vi "auto_alignment_v2-2.vi"() -> ()   [LabVIEW 2024]
uses:
  O:/DSG/Tyler/EIC/DIRC/daq/automated/Thorlabs.MotionControl.IntegratedStepperMotorsCLI.dll
  Thorlabs.MotionControl.IntegratedStepperMotorsCLI.dll
  O:/DSG/Tyler/EIC/DIRC/daq/automated/Thorlabs.MotionControl.Benchtop.StepperMotorCLI.dll
  Thorlabs.MotionControl.Benchtop.StepperMotorCLI.dll
  301acc45-ca86-4456-a934-959b204451cf.vi
  874d4c17-ce3d-4308-86ed-5be04f0cb30b.vi
  5035e5c4-651a-4bea-8586-5c5be43a7c01.vi
  c928da2b-9bf4-4dff-b90d-86dfb6fa8dbf.vi
  97e29fd1-0a36-40b5-96b6-4bface3040cf.vi
  <vilib>/Array/Sort 2D Array - Pop Stack.vi
  <vilib>/Array/Sort 2D Array - Push Stack.vi
  301acc45-ca86-4456-a934-959b204451cf.vi/269d4b3b-47f5-49e3-8884-44851e4dd9d5.vi
  301acc45-ca86-4456-a934-959b204451cf.vi/6d99389c-673d-4efb-bf33-19b32bcf4cf8.vi
  874d4c17-ce3d-4308-86ed-5be04f0cb30b.vi/269d4b3b-47f5-49e3-8884-44851e4dd9d5.vi
  874d4c17-ce3d-4308-86ed-5be04f0cb30b.vi/6d99389c-673d-4efb-bf33-19b32bcf4cf8.vi
  5035e5c4-651a-4bea-8586-5c5be43a7c01.vi/269d4b3b-47f5-49e3-8884-44851e4dd9d5.vi
  5035e5c4-651a-4bea-8586-5c5be43a7c01.vi/6d99389c-673d-4efb-bf33-19b32bcf4cf8.vi
  c928da2b-9bf4-4dff-b90d-86dfb6fa8dbf.vi/269d4b3b-47f5-49e3-8884-44851e4dd9d5.vi
  c928da2b-9bf4-4dff-b90d-86dfb6fa8dbf.vi/6d99389c-673d-4efb-bf33-19b32bcf4cf8.vi
  97e29fd1-0a36-40b5-96b6-4bface3040cf.vi/269d4b3b-47f5-49e3-8884-44851e4dd9d5.vi
  97e29fd1-0a36-40b5-96b6-4bface3040cf.vi/6d99389c-673d-4efb-bf33-19b32bcf4cf8.vi
  <vilib>/Utility/file.llb/Read Delimited Spreadsheet (string).vi
  <vilib>/Analysis/NI_AALBase.lvlib
panel:
  out "sim_y-range":dbl[](array[numeric])
  out "sim_x-range":dbl[](array[numeric])
  out "sim_max":dbl[](array[numeric])
  out "Array":string[](array[string])
  in  "early-stop":bool
  out "state":string
  out "nPts":dbl
  out "pt-history":dbl[][](array[numeric])
  out "real-mode":bool
  out "sim-iCorr":dbl[](array[numeric])
  out "sim-pdy":dbl[](array[numeric])
  out "sim-pdx":dbl[](array[numeric])
  out "sim-data":dbl[][](array[numeric])
  out "Final Location":dbl[](array[numeric])
  out "x_c":dbl[](array[numeric])
  out "x_e":dbl[](array[numeric])
  out "x_r":dbl[](array[numeric])
  out "timeout":bool
  out "se_done":bool
  in  "se_goal":dbl=0.04
  out "squared_error":dbl
  out "x_o":dbl[](array[numeric])
  in  "xStart":dbl=265.0 format="%#_13g"
  in  "yStart":dbl=127.5 format="%#_13g"
  in  "stage-refs":T1
  in  "nSamples":dbl=10.0 caption="# Samples"
  in  "NM-params":T2={"alpha"=1.0, "gamma"=2.0, "rho"=0.5, "sigma"=0.5, "simplex L"=0.5}
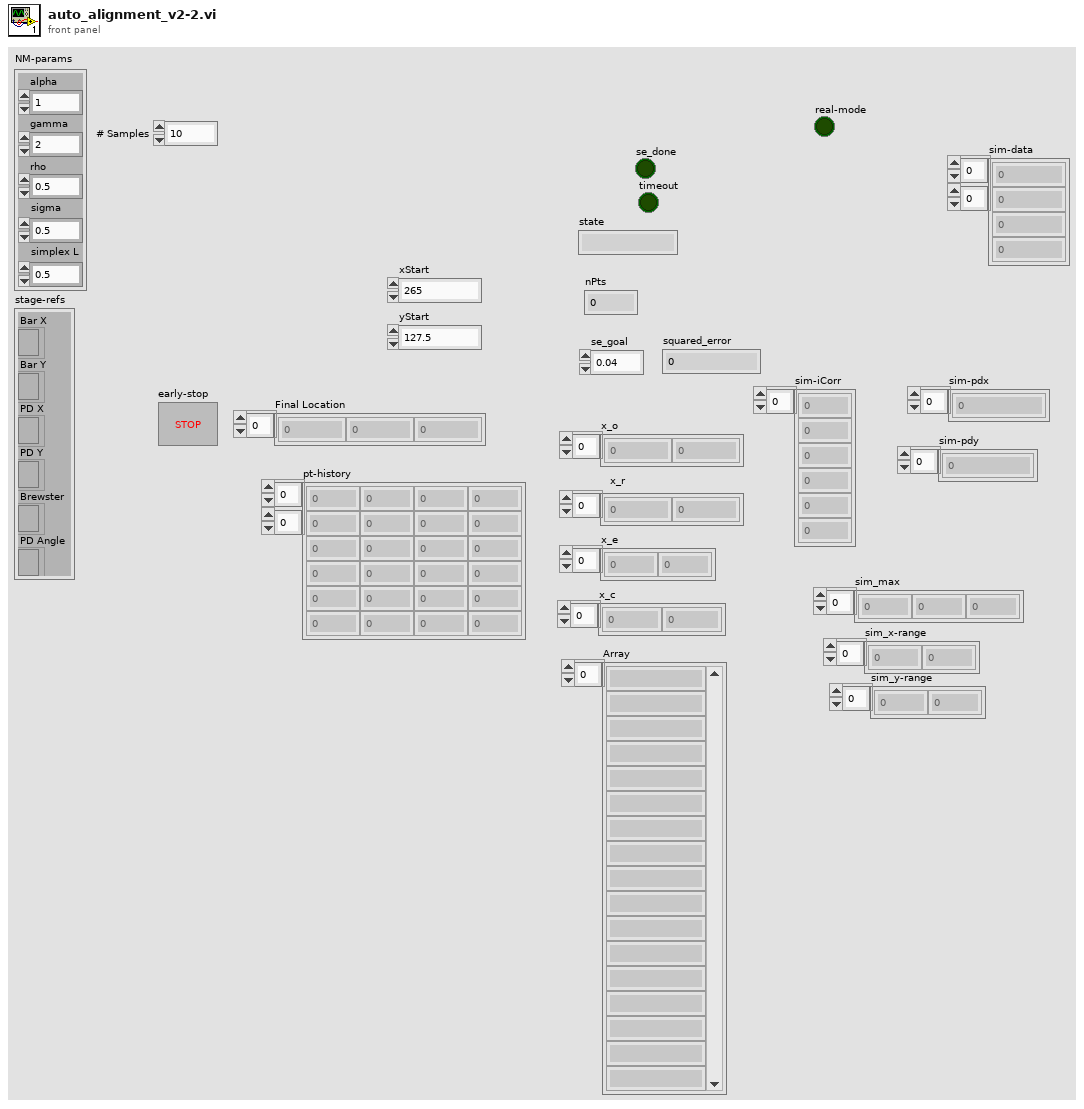
[diagram p1: front panel]
types:
  T1 = cluster{"Bar X":refnum<k24>, "Bar Y":refnum<k24>, "PD X":refnum<k24>, "PD Y":refnum<k24>, "Brewster":refnum<k24>, "PD Angle":refnum<k24>}
  T2 = cluster{"alpha":dbl, "gamma":dbl, "rho":dbl, "sigma":dbl, "simplex L":dbl}
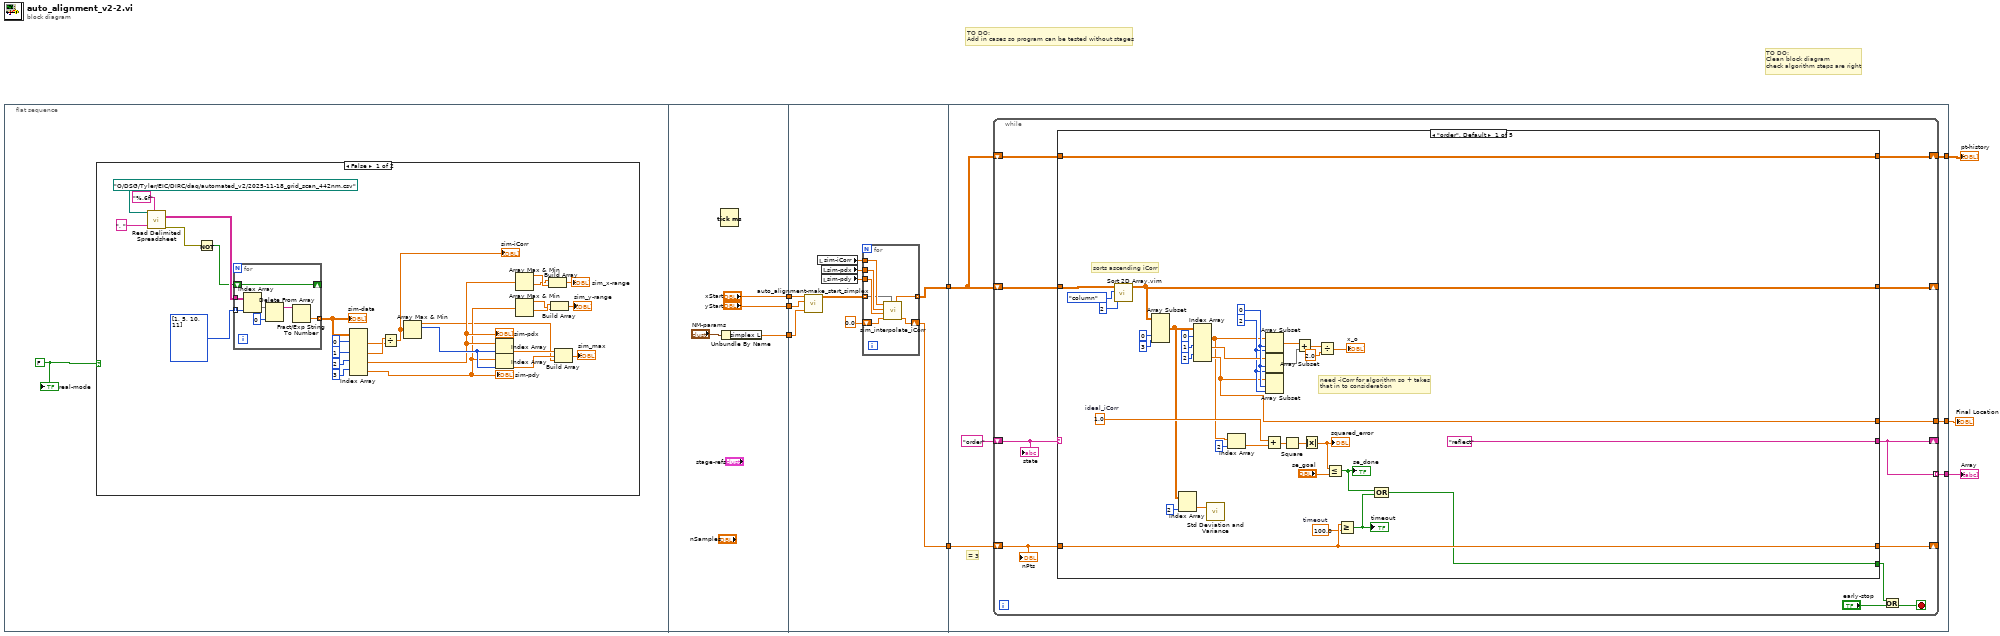
[diagram p0: block diagram]
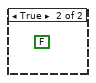
[diagram p2: hidden frame]
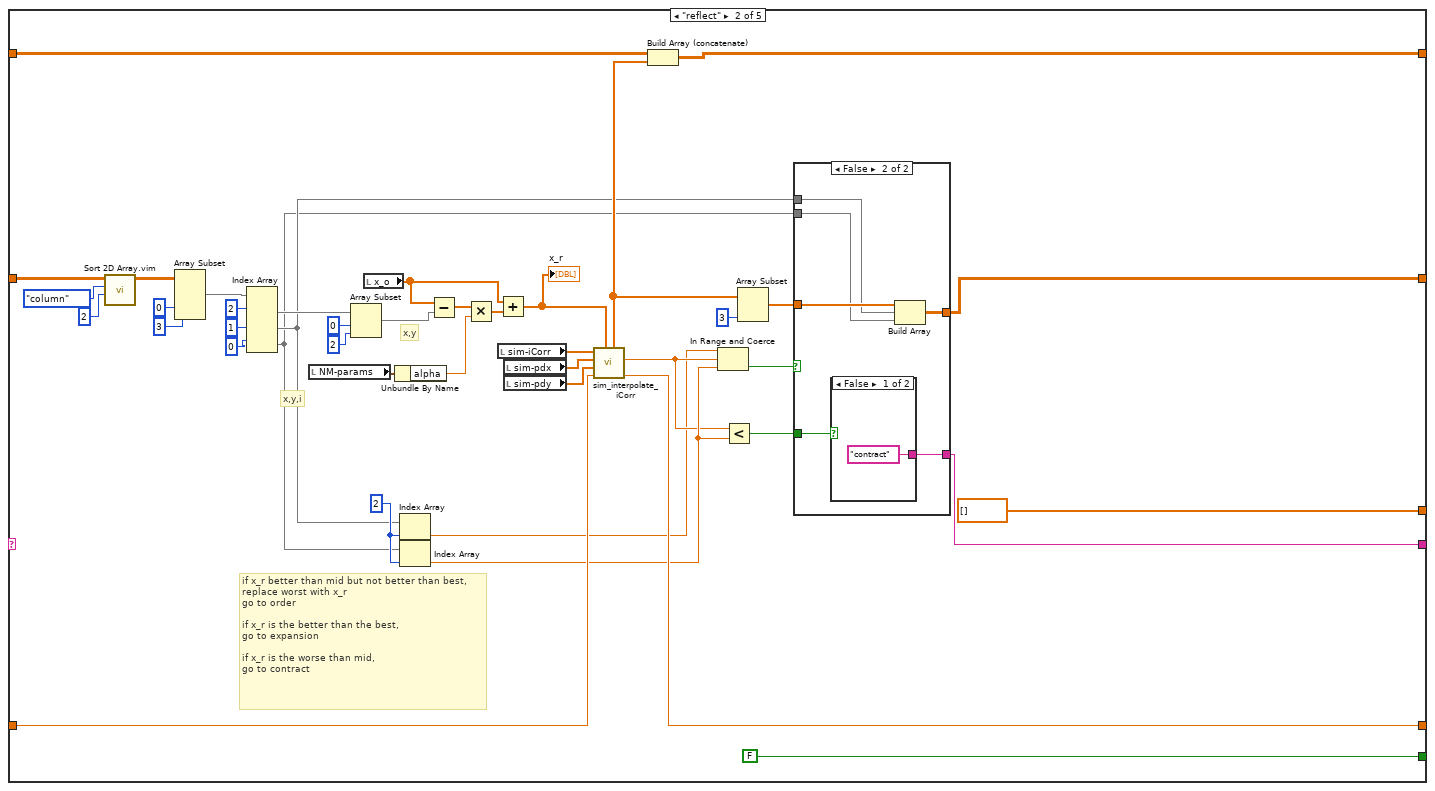
[diagram p3: hidden frame]
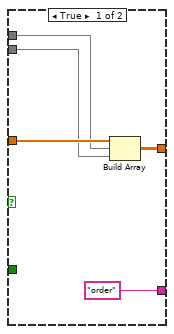
[diagram p4: hidden frame]
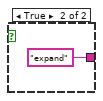
[diagram p5: hidden frame]
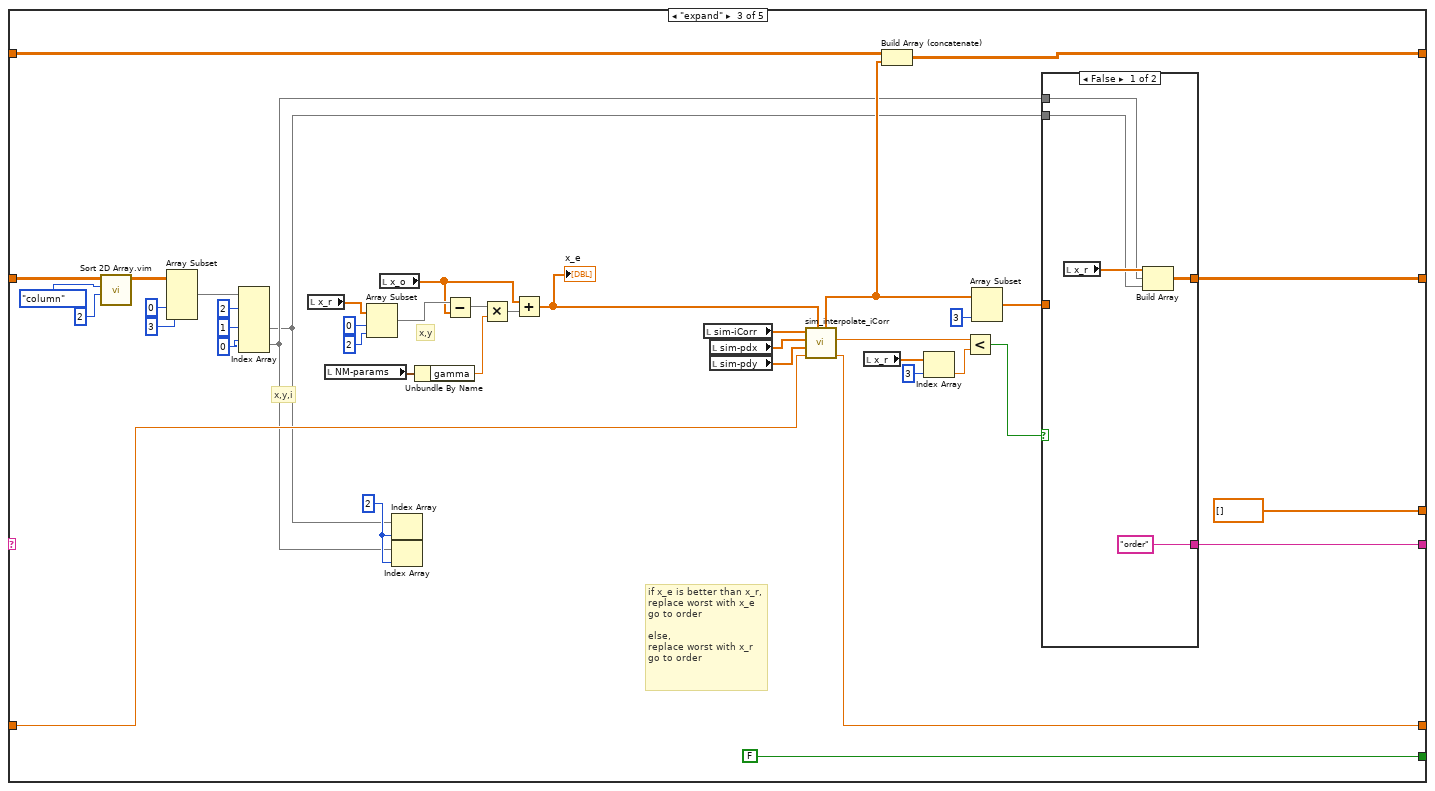
[diagram p6: hidden frame]
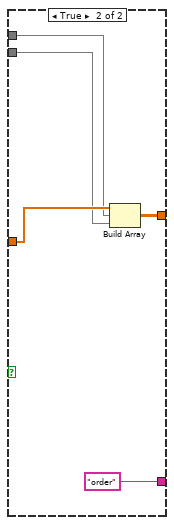
[diagram p7: hidden frame]
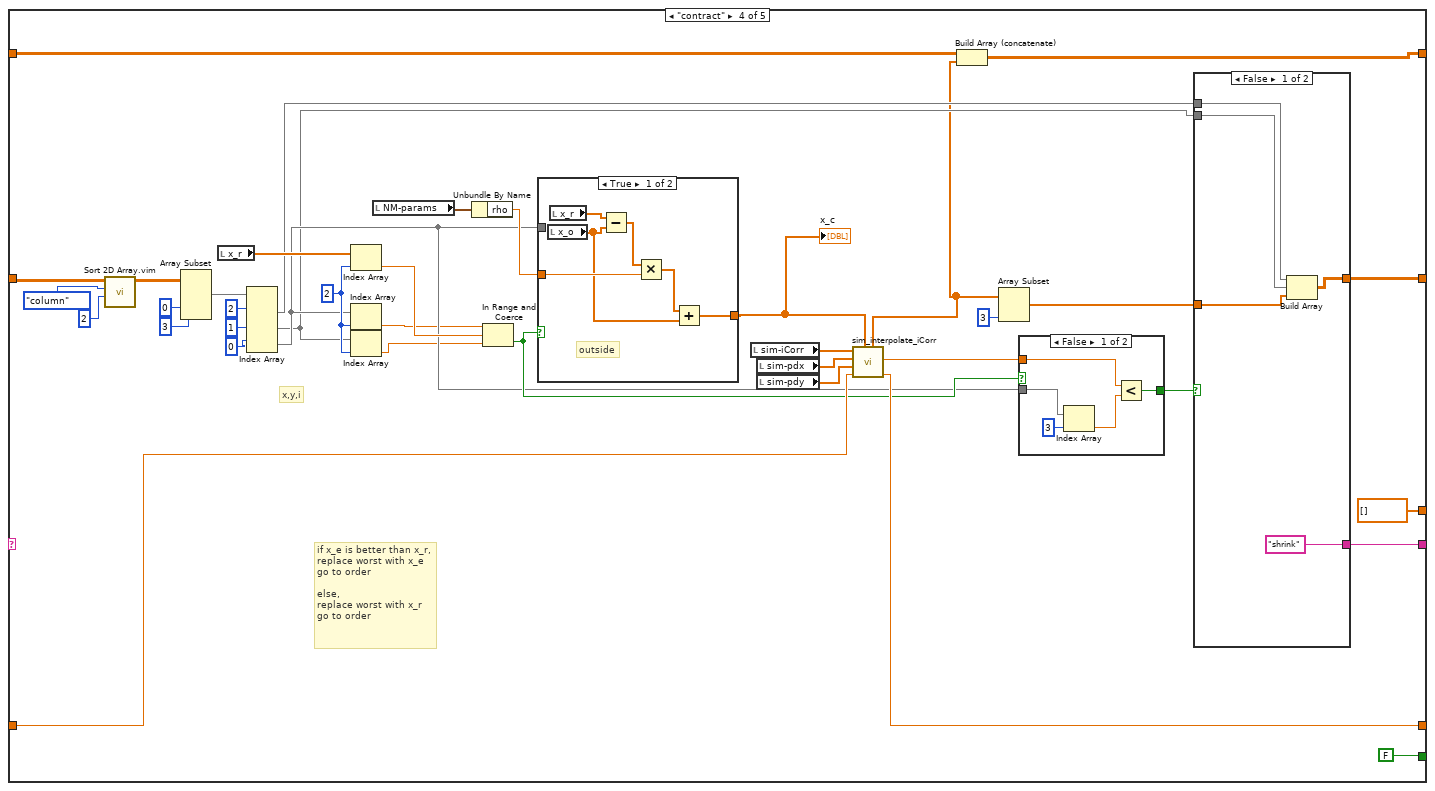
[diagram p8: hidden frame]
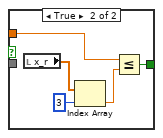
[diagram p9: hidden frame]
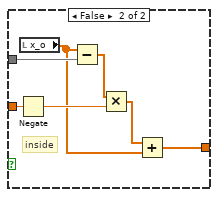
[diagram p10: hidden frame]
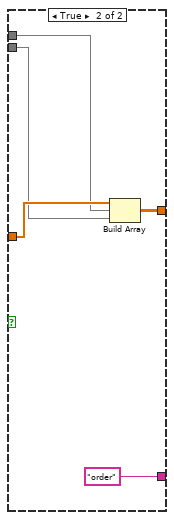
[diagram p11: hidden frame]
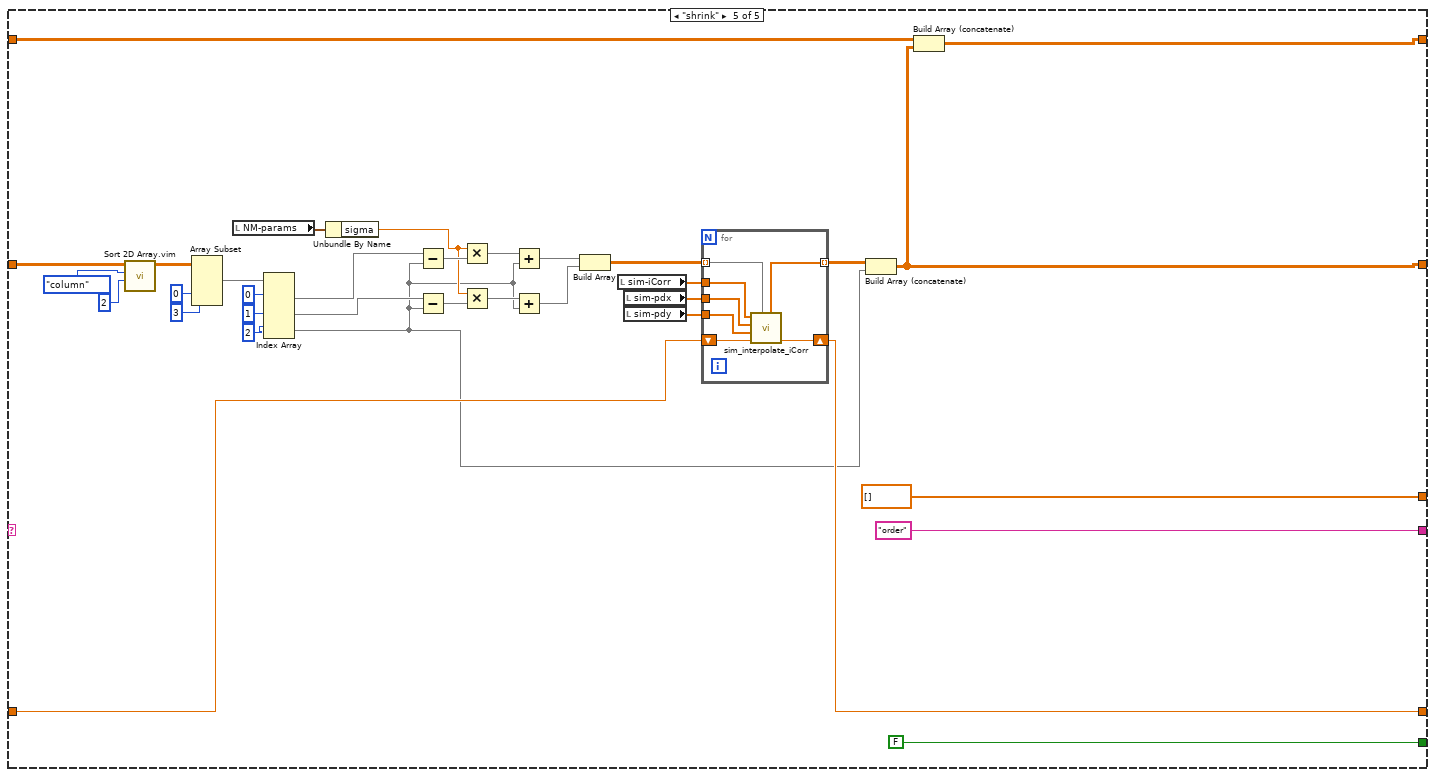
[diagram p12: hidden frame]
diagram:
  # "TO DO:\nClean block diagram\ncheck algorithm steps are right"
  # "TO DO:\nAdd in cases so program can be tested without stages"
  n1 = flat-sequence {
    tunnel: ["xStart"] -> w8
    tunnel: ["yStart"] -> w7
    tunnel: [w45] -> w6
    tunnel: [w58] -> w2
    tunnel: [w57] -> w1
    tunnel: w6 -> [w56]
    tunnel: w7 -> [w55]
    tunnel: w8 -> [w54]
    tunnel: w2 -> [w69]
    tunnel: w1 -> [w70]
    tunnel: [w68] -> w5
    tunnel: [w67] -> w4
    tunnel: [w66] -> w3
    frame #0 {
      w9 = FALSE
      n2 = case shown="False" w9 {
        frame False {
          n3 = call-poly <vilib>:"Read Delimited Spreadsheet.vi"("file path (dialog if empty)"=path "O:/DSG/Tyler/EIC/DIRC/daq/automated_v2/2025-11-18_grid_scan_442nm.csv", "format (%s)"="%.6f" ("format (%.3f)"), "delimiter (\\t)"=", " ("delimiter (\\t)")) -> ("all rows"=w33:string[][], "error out"=w35:errorcluster)  [unwired: 7 in, 4 out]
          n4 = Not(x=w35) -> (.not. x?=w31:bool)
          n5 = for {
            tunnel: i32[] [1, 5, 10, 11] -> [w43] mode=indexing
            tunnel: w33 -> [w44]
            shift-right: [w42] -> _
            shift-left: w31 -> [w42]
            tunnel: [w38] -> w24 mode=indexing
            n6 = Index Array(array=w44, index (col)=w43) -> (element=w41:string[])  [unwired: 1 in]
            n7 = Delete From Array(array=w41, index=0) -> (array with subset deleted=w39:string[])  [unwired: 1 in, 1 out]
            n8 = Fract/Exp String To Number(string=w39) -> (number=w38:dbl[])  [unwired: 3 in, 1 out]
          }
          "sim-data" <- w24
          n9 = Index Array(array=w24, index (row) #1=0 ("index"), index (row) #2=1 ("index (row)"), index (row) #3=2 ("index (row)"), index (row) #4=3 ("index (row)")) -> (element #1=w25:dbl[], element #2=w26:dbl[], element #3=w19:dbl[], element #4=w18:dbl[])  [unwired: 4 in]
          "sim-pdx" <- w19
          "sim-pdy" <- w18
          n10 = Divide(x=w26, y=w25) -> (x/y=w10:dbl[])
          "sim-iCorr" <- w10
          n11 = Array Max & Min(array=w10) -> (max value=w11:dbl, max index (indices)=w23:i32)  [unwired: 2 out]
          n12 = Index Array(array=w19, index=w23) -> (element=w22:dbl)
          n13 = Index Array(array=w18, index=w23) -> (element=w21:dbl)
          n14 = Array Max & Min(array=w19) -> (max value=w17:dbl, min value=w16:dbl)  [unwired: 2 out]
          n15 = Array Max & Min(array=w18) -> (max value=w13:dbl, min value=w15:dbl)  [unwired: 2 out]
          n16 = Build Array(w16, w17) -> (→"sim_x-range":dbl[])
          n17 = Build Array(w15, w13) -> (→"sim_y-range":dbl[])
          n18 = Build Array(w22, w21, w11) -> (→"sim_max":dbl[])
        }
        frame True {
          (unwired) FALSE
        }
      }
      "real-mode" <- w9
    }
    frame #1 {
      n19 = Tick Count (ms)() -> ()  [unwired: 1 out]
      n20 = Unbundle By Name("NM-params") -> ("simplex L"=w45:dbl)
    }
    frame #2 {
      n21 = call "auto_alignment-make_start_simplex.vi"("L"=w56, "yStart"=w55, "xStart"=w54) -> ("Array"=w53:dbl[][])  [unwired: 8 in]
      n22 = local read "sim-iCorr"() -> (w51:dbl[])
      n23 = local read "sim-pdx"() -> (w49:dbl[])
      n24 = local read "sim-pdy"() -> (w50:dbl[])
      n25 = for {
        shift-right: [w60] -> w57
        shift-left: 0.0 -> [w59]
        tunnel: w53 -> [w62] mode=indexing
        tunnel: [w61] -> w58 mode=indexing
        tunnel: w51 -> [w65]
        tunnel: w50 -> [w63]
        tunnel: w49 -> [w64]
        n26 = call "sim_interpolate_iCorr.vi"("point in"=w62, "nPts in"=w59, "sim-pdy"=w63, "sim-pdx"=w64, "sim-iCorr"=w65) -> ("nPts out"=w60:dbl, "measured-point out"=w61:dbl[])  [unwired: 4 in, 1 out]
      }
    }
    frame #3 {
      # "= 3"
      n27 = while {
        shift-right: [w77] -> w67
        shift-left: w69 -> [w82]
        shift-right: [w78] -> _
        shift-left: w69 -> [w81]
        shift-right: [w72] -> _
        shift-left: "order" -> [w83]
        shift-right: [w79] -> _
        shift-left: w70 -> [w80]
        tunnel: [w76] -> w68
        tunnel: [w72] -> w66 mode=indexing
        stop <- w74 stop-if-true
        n28 = case shown="\"order\", Default" w83 {
          tunnel: w82 -> [w105 w143 w200 w254 w311]
          tunnel: w81 -> [w104 w121 w176 w229 w298]
          tunnel: ["reflect" w139 w196 w251 "order"] -> w72
          tunnel: w80 -> [w95 w145 w202 w256 w312]
          tunnel: [w95 w144 w201 w255 w309] -> w79
          tunnel: [w96 w140 w197 w252 w306] -> w78
          tunnel: [w91 FALSE FALSE FALSE FALSE] -> w73
          tunnel: [w105 w142 w199 w253 w310] -> w77
          tunnel: [w90 dbl[] [] dbl[] [] dbl[] [] dbl[] []] -> w76
          frame "order", Default {
            w94 = 100.0  # timeout
            w101 = 1.0  # ideal_iCorr
            w110 = 2 ("length")
            w112 = 0 ("index")
            # "need -iCorr for algorithm so + takes\nthat in to consideration"
            # "sorts ascending iCorr"
            n29 = call "Sort 2D Array.vim"("index"=2, "dimension to index (column)"=enum16{"column", "row"}."column", "2D array"=w104) -> ("sorted 2D array"=w96:dbl[][])  [unwired: 7 in, 1 out]
            n30 = Array Subset(array=w96, index (col)=0 ("index"), length (col)=3 ("length")) -> (w86:dbl[][])  [unwired: 2 in]
            n31 = Index Array(array=w86, index (col)=2 ("disabled index (col)")) -> (element=w84:dbl[])  [unwired: 1 in]
            n32 = Index Array(array=w86, index (row) #1=0 ("index (row)"), index (row) #2=1 ("index (row)"), index (row) #3=2 ("index (row)")) -> (element #1=w87:dbl[], element #2=w111:dbl[], element #3=w90:dbl[])  [unwired: 3 in]
            n33 = call <vilib>:"Std Deviation and Variance.vi"("X"=w84) -> ()  [unwired: 1 in, 3 out]
            n34 = Index Array(array=w87, index=2) -> (element=w102:dbl)
            n35 = Add(x=w101, y=w102) -> (x+y=w100:dbl)
            n36 = Array Subset(array=w87, index=w112, length=w110) -> (w89:dbl[])
            n37 = Array Subset(array=w111, index=w112, length=w110) -> (w88:dbl[])
            n38 = Array Subset(array=w90, index=w112, length=w110) -> ()  [unwired: 1 out]
            n39 = Square(x=w100) -> (x^2=w99:dbl)
            n40 = Add(x=w89, y=w88) -> (x+y=w109:dbl[])
            n41 = Absolute Value(x=w99) -> (abs(x)=w98:dbl)
            "squared_error" <- w98
            n42 = Divide(x=w109, y=2.0) -> (x/y=→"x_o":dbl[])
            n43 = Less Or Equal?(x=w98, y="se_goal") -> (x <= y?=w93:bool)
            "se_done" <- w93
            n44 = Greater Or Equal?(x=w95, y=w94) -> (x >= y?=w92:bool)
            "timeout" <- w92
            n45 = Compound Arithmetic op=OR(w93, w92) -> (w91:bool)
          }
          frame "reflect" {
            w141 = 2 ("index")
            # "x,y"
            # "if x_r better than mid but not better than best, \nreplace worst with x_r\ngo to order\n\nif x_r is the better than the best,\ngo to expansion\n\nif x_r is the worse than mid,\ngo to contract"
            # "x,y,i"
            n46 = call "Sort 2D Array.vim"("index"=2, "dimension to index (column)"=enum16{"column", "row"}."column", "2D array"=w121) -> ("sorted 2D array"=w120:dbl[][])  [unwired: 7 in, 1 out]
            n47 = Array Subset(array=w120, index (col)=0 ("index"), length (col)=3 ("length")) -> (w129:dbl[][])  [unwired: 2 in]
            n48 = Index Array(array=w129, index (row) #1=2 ("index (row)"), index (row) #2=1 ("index (row)"), index (row) #3=0 ("index (row)")) -> (element #1=w155:dbl[], element #2=w128:dbl[], element #3=w127:dbl[])  [unwired: 3 in]
            n49 = local read "NM-params"() -> (w152:T2)
            n50 = Array Subset(array=w155, index=0 ("index (row)"), length=2 ("index (row)")) -> (w151:dbl[])
            n51 = local read "x_o"() -> (w148:dbl[])
            n52 = Unbundle By Name(w152) -> ("alpha"=w149:dbl)
            n53 = Index Array(array=w128, index=w141) -> (element=w131:dbl)
            n54 = Index Array(array=w127, index=w141) -> (element=w134:dbl)
            n55 = Subtract(x=w148, y=w151) -> (x-y=w150:dbl[])
            n56 = Multiply(x=w150, y=w149) -> (x*y=w147:dbl[])
            n57 = Add(x=w148, y=w147) -> (x+y=w146:dbl[])
            "x_r" <- w146
            n58 = local read "sim-iCorr"() -> (w126:dbl[])
            n59 = local read "sim-pdx"() -> (w125:dbl[])
            n60 = local read "sim-pdy"() -> (w124:dbl[])
            n61 = call "sim_interpolate_iCorr.vi"("point in"=w146, "nPts in"=w145, "sim-pdy"=w124, "sim-pdx"=w125, "sim-iCorr"=w126) -> ("nPts out"=w144:dbl, "iCorr out"=w132:dbl, "measured-point out"=w138:dbl[])  [unwired: 4 in]
            n62 = Build Array (concatenate)(w143, w138) -> (w142:dbl[][])
            n63 = In Range and Coerce(upper limit=w131, x=w132, lower limit=w134) -> (In Range?=w133:bool)  [unwired: 1 out]
            n64 = Less?(x=w132, y=w134) -> (x < y?=w130:bool)
            n65 = Array Subset(array=w138, length=3) -> (w136:dbl[])  [unwired: 1 in]
            n66 = case shown="False" w133 {
              tunnel: [w165 w170] -> w140
              tunnel: ["order" w172] -> w139
              tunnel: w136 -> [w166 w169]
              tunnel: w130 -> [_ w171]
              tunnel: w128 -> [w163 w168]
              tunnel: w127 -> [w162 w167]
              frame True {
                n67 = Build Array(w166, w163, w162) -> (w165:dbl[][])
              }
              frame False {
                n68 = case shown="False" w171 {
                  tunnel: ["contract" "expand"] -> w172
                  frame False {
                  }
                  frame True {
                  }
                }
                n69 = Build Array(w169, w168, w167) -> (w170:dbl[][])
              }
            }
          }
          frame "expand" {
            w198 = 2 ("index")
            # "x,y"
            # "if x_e is better than x_r,\nreplace worst with x_e\ngo to order\n\nelse,\nreplace worst with x_r\ngo to order"
            # "x,y,i"
            n70 = call "Sort 2D Array.vim"("index"=2, "dimension to index (column)"=enum16{"column", "row"}."column", "2D array"=w176) -> ("sorted 2D array"=w175:dbl[][])  [unwired: 7 in, 1 out]
            n71 = Array Subset(array=w175, index (col)=0 ("index"), length (col)=3 ("length")) -> (w215:dbl[][])  [unwired: 2 in]
            n72 = Index Array(array=w215, index (row) #1=2 ("index (row)"), index (row) #2=1 ("index (row)"), index (row) #3=0 ("index (row)")) -> (element #2=w182:dbl[], element #3=w183:dbl[])  [unwired: 3 in, 1 out]
            n73 = local read "x_r"() -> (w192:dbl[])
            n74 = local read "NM-params"() -> (w207:T2)
            n75 = Array Subset(array=w192, index=0 ("index (row)"), length=2 ("index (row)")) -> (w185:dbl[])
            n76 = local read "x_o"() -> (w184:dbl[])
            n77 = Index Array(array=w182, index=w198) -> ()  [unwired: 1 out]
            n78 = Index Array(array=w183, index=w198) -> ()  [unwired: 1 out]
            n79 = Unbundle By Name(w207) -> ("gamma"=w205:dbl)
            n80 = Subtract(x=w185, y=w184) -> (x-y=w206:dbl[])
            n81 = Multiply(x=w206, y=w205) -> (x*y=w204:dbl[])
            n82 = Add(x=w184, y=w204) -> (x+y=w203:dbl[])
            "x_e" <- w203
            n83 = local read "sim-iCorr"() -> (w181:dbl[])
            n84 = local read "sim-pdx"() -> (w180:dbl[])
            n85 = local read "sim-pdy"() -> (w179:dbl[])
            n86 = call "sim_interpolate_iCorr.vi"("point in"=w203, "nPts in"=w202, "sim-pdy"=w179, "sim-pdx"=w180, "sim-iCorr"=w181) -> ("nPts out"=w201:dbl, "iCorr out"=w190:dbl, "measured-point out"=w195:dbl[])  [unwired: 4 in]
            n87 = local read "x_r"() -> (w189:dbl[])
            n88 = Build Array (concatenate)(w200, w195) -> (w199:dbl[][])
            n89 = Index Array(array=w189, index=3) -> (element=w187:dbl)
            n90 = Less?(x=w190, y=w187) -> (x < y?=w191:bool)
            n91 = Array Subset(array=w195, length=3) -> (w193:dbl[])  [unwired: 1 in]
            n92 = case shown="False" w191 {
              tunnel: [w221 w225] -> w197
              tunnel: ["order" "order"] -> w196
              tunnel: w193 -> [_ w226]
              tunnel: w183 -> [w218 w223]
              tunnel: w182 -> [w217 w222]
              frame False {
                n93 = local read "x_r"() -> (w219:dbl[])
                n94 = Build Array(w219, w218, w217) -> (w221:dbl[][])
              }
              frame True {
                n95 = Build Array(w226, w223, w222) -> (w225:dbl[][])
              }
            }
          }
          frame "contract" {
            w248 = 2 ("index")
            # "if x_e is better than x_r,\nreplace worst with x_e\ngo to order\n\nelse,\nreplace worst with x_r\ngo to order"
            # "x,y,i"
            n96 = call "Sort 2D Array.vim"("index"=2, "dimension to index (column)"=enum16{"column", "row"}."column", "2D array"=w229) -> ("sorted 2D array"=w227:dbl[][])  [unwired: 7 in, 1 out]
            n97 = Array Subset(array=w227, index (col)=0 ("index"), length (col)=3 ("length")) -> (w263:dbl[][])  [unwired: 2 in]
            n98 = local read "x_r"() -> (w246:dbl[])
            n99 = Index Array(array=w263, index (row) #1=2 ("index (row)"), index (row) #2=1 ("index (row)"), index (row) #3=0 ("index (row)")) -> (element #1=w237:dbl[], element #2=w236:dbl[], element #3=w242:dbl[])  [unwired: 3 in]
            n100 = Index Array(array=w246, index=w248) -> (element=w247:dbl)
            n101 = Index Array(array=w242, index=w248) -> (element=w240:dbl)
            n102 = Index Array(array=w236, index=w248) -> (element=w241:dbl)
            n103 = local read "NM-params"() -> (w257:T2)
            n104 = Unbundle By Name(w257) -> ("rho"=w245:dbl)
            n105 = In Range and Coerce(upper limit=w240, x=w247, lower limit=w241) -> (In Range?=w244:bool)  [unwired: 1 out]
            n106 = case shown="True" w244 {
              tunnel: w245 -> [w278 w286]
              tunnel: [w275 w284] -> w232
              tunnel: w242 -> [_ w283]
              frame True {
                # "outside"
                n107 = local read "x_o"() -> (w276:dbl[])
                n108 = local read "x_r"() -> (w280:dbl[])
                n109 = Subtract(x=w280, y=w276) -> (x-y=w279:dbl[])
                n110 = Multiply(x=w279, y=w278) -> (x*y=w277:dbl[])
                n111 = Add(x=w277, y=w276) -> (x+y=w275:dbl[])
              }
              frame False {
                # "inside"
                n112 = Negate(x=w286) -> (-x=w282:dbl)
                n113 = local read "x_o"() -> (w281:dbl[])
                n114 = Subtract(x=w281, y=w283) -> (x-y=w287:dbl[])
                n115 = Multiply(x=w287, y=w282) -> (x*y=w285:dbl[])
                n116 = Add(x=w285, y=w281) -> (x+y=w284:dbl[])
              }
            }
            "x_c" <- w232
            n117 = local read "sim-iCorr"() -> (w235:dbl[])
            n118 = local read "sim-pdx"() -> (w234:dbl[])
            n119 = local read "sim-pdy"() -> (w233:dbl[])
            n120 = call "sim_interpolate_iCorr.vi"("point in"=w232, "nPts in"=w256, "sim-pdy"=w233, "sim-pdx"=w234, "sim-iCorr"=w235) -> ("nPts out"=w255:dbl, "iCorr out"=w239:dbl, "measured-point out"=w231:dbl[])  [unwired: 4 in]
            n121 = Build Array (concatenate)(w254, w231) -> (w253:dbl[][])
            n122 = Array Subset(array=w231, length=3) -> (w249:dbl[])  [unwired: 1 in]
            n123 = case shown="False" w244 {
              tunnel: w242 -> [w268 _]
              tunnel: w239 -> [w266 w272]
              tunnel: [w267 w270] -> w238
              frame False {
                n124 = Index Array(array=w268, index=3) -> (element=w265:dbl)
                n125 = Less?(x=w266, y=w265) -> (x < y?=w267:bool)
              }
              frame True {
                n126 = local read "x_r"() -> (w273:dbl[])
                n127 = Index Array(array=w273, index=3) -> (element=w271:dbl)
                n128 = Less Or Equal?(x=w272, y=w271) -> (x <= y?=w270:bool)
              }
            }
            n129 = case shown="False" w238 {
              tunnel: [w291 w296] -> w252
              tunnel: ["shrink" "order"] -> w251
              tunnel: w249 -> [w290 w297]
              tunnel: w237 -> [w289 w294]
              tunnel: w236 -> [w288 w293]
              frame False {
                n130 = Build Array(w289, w288, w290) -> (w291:dbl[][])
              }
              frame True {
                n131 = Build Array(w297, w294, w293) -> (w296:dbl[][])
              }
            }
          }
          frame "shrink" {
            n132 = call "Sort 2D Array.vim"("index"=2, "dimension to index (column)"=enum16{"column", "row"}."column", "2D array"=w298) -> ("sorted 2D array"=w299:dbl[][])  [unwired: 7 in, 1 out]
            n133 = Array Subset(array=w299, index (col)=0 ("index"), length (col)=3 ("length")) -> (w329:dbl[][])  [unwired: 2 in]
            n134 = local read "NM-params"() -> (w323:T2)
            n135 = Index Array(array=w329, index (row) #1=0 ("index (row)"), index (row) #2=1 ("index (row)"), index (row) #3=2 ("index (row)")) -> (element #1=w322:dbl[], element #2=w318:dbl[], element #3=w305:dbl[])  [unwired: 3 in]
            n136 = Unbundle By Name(w323) -> ("sigma"=w319:dbl)
            n137 = Subtract(x=w322, y=w305) -> (x-y=w320:dbl[])
            n138 = Subtract(x=w318, y=w305) -> (x-y=w321:dbl[])
            n139 = Multiply(x=w319, y=w320) -> (x*y=w317:dbl[])
            n140 = Multiply(x=w319, y=w321) -> (x*y=w316:dbl[])
            n141 = Add(x=w317, y=w305) -> (x+y=w315:dbl[])
            n142 = Add(x=w316, y=w305) -> (x+y=w314:dbl[])
            n143 = Build Array(w315, w314) -> (w313:dbl[][])
            n144 = local read "sim-iCorr"() -> (w304:dbl[])
            n145 = local read "sim-pdx"() -> (w303:dbl[])
            n146 = local read "sim-pdy"() -> (w302:dbl[])
            n147 = for {
              shift-right: [w333] -> w309
              shift-left: w312 -> [w332]
              tunnel: w313 -> [w335] mode=indexing
              tunnel: [w334] -> w308 mode=indexing
              tunnel: w304 -> [w338]
              tunnel: w303 -> [w337]
              tunnel: w302 -> [w336]
              n148 = call "sim_interpolate_iCorr.vi"("point in"=w335, "nPts in"=w332, "sim-pdy"=w336, "sim-pdx"=w337, "sim-iCorr"=w338) -> ("nPts out"=w333:dbl, "measured-point out"=w334:dbl[])  [unwired: 4 in, 1 out]
            }
            n149 = Build Array (concatenate)(w308, w305) -> (w306:dbl[][])
            n150 = Build Array (concatenate)(w311, w306) -> (w310:dbl[][])
          }
        }
        n151 = Or(x=w73, y="early-stop") -> (x .or. y?=w74:bool)
        "nPts" <- w80
        "state" <- w83
      }
    }
  }
  "Final Location" <- w5
  "pt-history" <- w4
  "Array" <- w3
